vi "Test DUT Self Test Triggers Self Test Broadcast Message.vi"(8 "error in (no error)":errorcluster, 11 "Device Under Test Test In":refnum<class "Device Under Test Test.lvclass">) -> (0 "error out":errorcluster, 3 "Device Under Test Test Out":refnum<class "Device Under Test Test.lvclass">)   [LabVIEW 2020, in "Device Under Test Test.lvclass"]
uses:
  Device Under Test Test.lvclass
  C:/Program Files (x86)/National Instruments/LabVIEW 2020/vi.lib/Astemes/LUnit/Test Case.lvclass
  Device Under Test/Device Under Test.lvclass
  C:/Program Files (x86)/National Instruments/LabVIEW 2020/vi.lib/Astemes/Triarc Framework/Process/Process.lvclass
  <vilib>/Astemes/Triarc Framework/Process/Process.lvclass/Process.ctl
  <vilib>/Astemes/LUnit/Test Case.lvclass/Test Case.ctl
  <vilib>/Astemes/Triarc Framework/Process/Public/Lifecycle/Get Lifecycle State.vi
  <vilib>/Astemes/Triarc Framework/Broadcast Event Helpers/Execution timer.vi
  <vilib>/Astemes/Triarc Framework/Process/Private/SubVIs/Wait for finish.vi
  <vilib>/Astemes/Triarc Framework/Process/Private/SubVIs/Set Lifecycle State.vi
  <vilib>/Astemes/Triarc Framework/Process/Protected/Messaging/Send Message.vi
  <vilib>/Astemes/LUnit/Set Assertion Type.vi
  <vilib>/Astemes/LUnit/Palette/Pass.vi
  <vilib>/Astemes/LUnit/Palette/Fail.vi
  <vilib>/Utility/error.llb/Clear Errors.vi
  <vilib>/Astemes/Triarc Framework/Process/Private/SubVIs/Handle Debug Data.vi
  <vilib>/Astemes/LUnit/Add test result.vi
  <vilib>/Utility/High Resolution Relative Seconds.vi
  <vilib>/Astemes/LUnit/LUnit Record Assertion Result.vi
  <vilib>/Astemes/LUnit/LUnit Aggregate Assertion Results.vi
  <vilib>/Astemes/LUnit/Method Result/LUnit Merge Status.vi
  <vilib>/Astemes/LUnit/LUnit Concatenate result strings.vi
  <vilib>/Utility/error.llb/Error Cluster From Error Code.vi
  <vilib>/Astemes/Triarc Framework/Broadcast Event Helpers/Dequeue Broadcast Message.vi
  <vilib>/Astemes/Triarc Framework/Process/Process.lvclass
  <vilib>/Astemes/LUnit/Test Case.lvclass
  <vilib>/Astemes/Triarc Framework/Broadcast Event Helpers/Broadcast Event Helpers.lvlib
panel:
  out "Message Data":variant
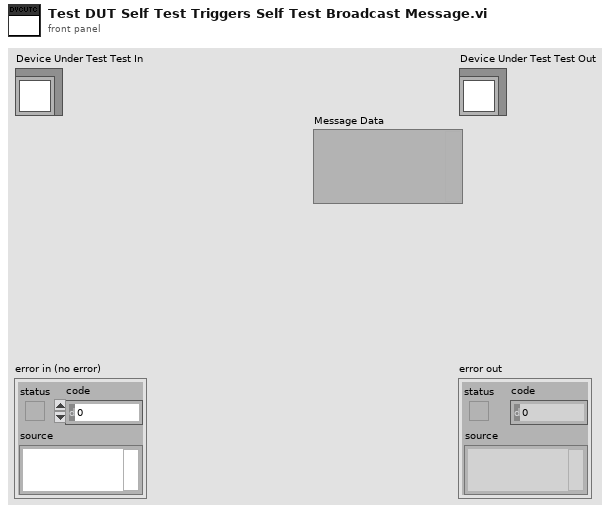
[diagram p1: front panel]
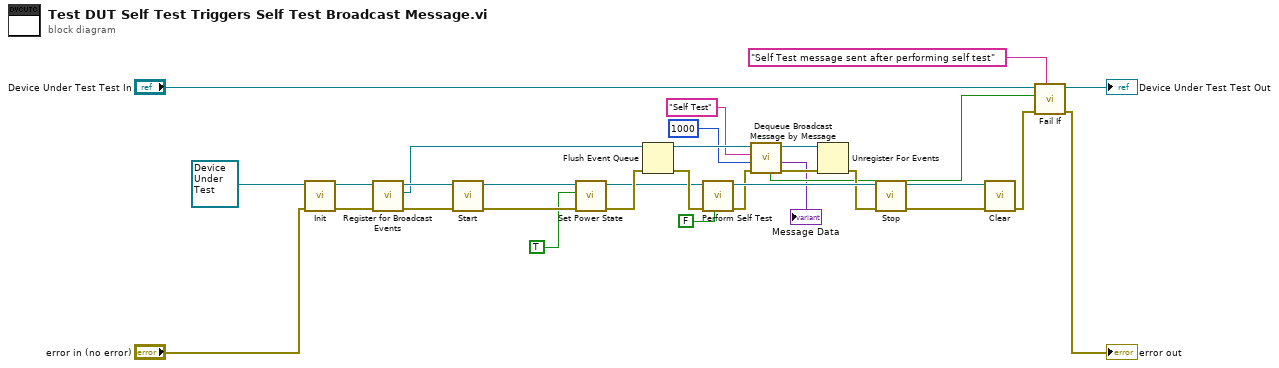
[diagram p0: block diagram]
diagram:
  n1 = call-dynamic "Init.vi"("error in (no error)"="error in (no error)", "View In"=refnum<class "Device Under Test.lvclass"> refnum ("Device Under Test.lvclass")) -> ("error out"=w23:errorcluster, "View Out"=w25:refnum<class "Device Under Test.lvclass">)  [unwired: 8 in]
  n2 = call <vilib>:"Register for Broadcast Events.vi"("error in (no error)"=w23, "Process In"=w25) -> ("error out"=w22:errorcluster, "Event Registration Refnum Out"=w12:refnum<event-registration>, "Process Out"=w24:refnum<class "Device Under Test.lvclass">)  [unwired: 7 in]
  n3 = call <vilib>:"Start.vi"("error in (no error)"=w22, "Process In"=w24) -> ("error out"=w30:errorcluster, "Process Out"=w5:refnum<class "Device Under Test.lvclass">)  [unwired: 7 in, 1 out]
  n4 = call "Set Power State.vi"("error in (no error)"=w30, "Power State"=TRUE, "Device Under Test In"=w5) -> ("error out"=w6:errorcluster, "Device Under Test Out"=w4:refnum<class "Device Under Test.lvclass">)  [unwired: 7 in]
  n5 = Flush Event Queue(0:w12, 3:w6) -> (8:w11:refnum<event-registration>, 11:w13:errorcluster)  [unwired: 4 in, 1 out]
  n6 = call "Perform Self Test.vi"("Wait for Reply?"=FALSE, "error in (no error)"=w13, "Device Under Test In"=w4) -> ("error out"=w15:errorcluster, "Device Under Test Out"=w29:refnum<class "Device Under Test.lvclass">)  [unwired: 5 in, 2 out]
  n7 = call <vilib>:"Dequeue Broadcast Message by Message.vi"("error in (no error)"=w15, "Timeout (-1)"=1000, "Message"="Self Test", "Event Registration Refnum"=w11) -> ("error out"=w14:errorcluster, "Message Data"=→"Message Data":variant, "Event Registration Refnum Out"=w9:refnum<event-registration>, "Timed Out?"=w7:bool)  [unwired: 3 in, 1 out]
  n8 = Unregister For Events(event registration refnum=w9, error in=w14) -> (error out=w10:errorcluster)
  n9 = call <vilib>:"Stop.vi"("error in (no error)"=w10, "Process In"=w29) -> ("error out"=w27:errorcluster, "Process Out"=w28:refnum<class "Device Under Test.lvclass">)  [unwired: 7 in, 1 out]
  n10 = call-dynamic "Clear.vi"("error in (no error)"=w27, "View In"=w28) -> ("error out"=w20:errorcluster)  [unwired: 9 in]
  n11 = call <vilib>:"Fail If.vi"("Description"="Self Test message sent after performing self test", "error in (no error)"=w20, "Fail?"=w7, "LUnit Test Case In"="Device Under Test Test In") -> ("error out"=→"error out":errorcluster, "LUnit Test Case Out"=→"Device Under Test Test Out":refnum<class "Device Under Test Test.lvclass">)  [unwired: 6 in]
